vi "Out_On_N4_201.vi"(4 "Driver Name":T8, 6 "Error Code":T9, 7 "ADJUST":T6, 8 "error in":T7, 11 "DriverConnect in":T1={"InterfaceType"=enum."VISA", "OpenedSession"="", "InterfaceSettings"={"Interface"=enum."RS232", "EOS 4 read"=enum."LF (\\n)", "EOS 4 write"=enum."LF (\\n)", "TMO, ms"=10000, "Sett"=variant(cluster{"Baud Rate":u32, "Data Bits":u16, "Parity":u16, "Stop Bits":u16, "Flow Control":u16, "Eho":bool} {"Baud Rate"=75, "Data Bits"=0, "Parity"=0, "Stop Bits"=0, "Flow Control"=0, "Eho"=FALSE})}}) -> (0 "error out":T7, 3 "DriverConnect out":T1={"InterfaceType"=enum."VISA", "OpenedSession"="", "InterfaceSettings"={"Interface"=enum."RS232", "EOS 4 read"=enum."LF (\\n)", "EOS 4 write"=enum."LF (\\n)", "TMO, ms"=10000, "Sett"=variant(cluster{"Baud Rate":u32, "Data Bits":u16, "Parity":u16, "Stop Bits":u16, "Flow Control":u16, "Eho":bool} {"Baud Rate"=75, "Data Bits"=0, "Parity"=0, "Stop Bits"=0, "Flow Control"=0, "Eho"=FALSE})}})   [LabVIEW 2018]
uses:
  MOKO_LabViewLibrary/MokoLowLevel/MokoLowLovelControl/MLLC_ErrorCode.ctl
  MOKO_LabViewLibrary/MokoLowLevel/MokoLowLovelControl/MLLC_DriverName.ctl
  MOKO_LabViewLibrary/MokoLowLevel/MokoLowLovelControl/MLLC_Error.ctl
  MOKO_LabViewLibrary/MokoLowLevel/MokoLowLovelControl/MLLC_Delay.ctl
  MOKO_LabViewLibrary/MokoLowLevel/MokoLowLovelControl/MLLC_ConnectCluster.ctl
  MOKO_LabViewLibrary/MokoLowLevel/MokoLowLovelControl/MLLC_InterfaceType.ctl
  MOKO_LabViewLibrary/MokoLowLevel/MokoLowLovelControl/MLLC_OpenedSession.ctl
  MOKO_LabViewLibrary/MokoLowLevel/MokoLowLovelControl/MLLC_InterfaceSettings.ctl
  MOKO_LabViewLibrary/MokoLowLevel/MokoLowLovelControl/MLLC_InterfaceKind.ctl
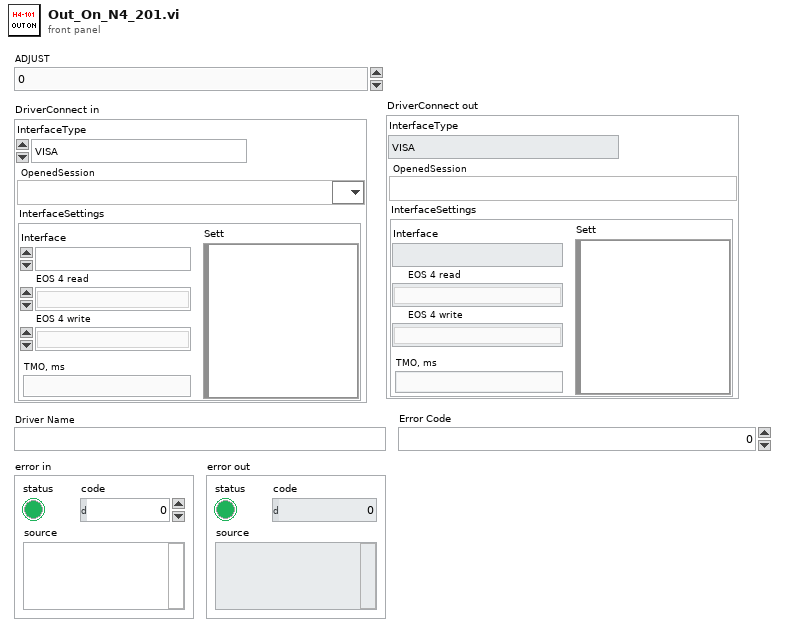
[diagram p1: front panel]
types:
  T1 = typedef "MLLC_ConnectCluster.ctl" = cluster{"InterfaceType":T2, "OpenedSession":T3, "InterfaceSettings":T4}
  T2 = typedef "MLLC_InterfaceType.ctl" = enum16{"VISA", "Prologix USB-GPIB"}
  T3 = typedef "MLLC_OpenedSession.ctl" = refnum<visa-resource-name>
  T4 = typedef "MLLC_InterfaceSettings.ctl" = cluster{"Interface":T5, "EOS 4 read":enum16{"Default (=EOS 4 write)", "CR (\\r)", "LF (\\n)", "None"}, "EOS 4 write":enum16{"CR+LF (\\r\\n)", "CR (\\r)", "LF (\\n)", "None"}, "TMO, ms":i32, "Sett":variant}
  T5 = typedef "MLLC_InterfaceKind.ctl" = enum16{"RS232", "GPIB", "USB", "Ethernet", "another"}
  T6 = typedef "MLLC_Delay.ctl" = dbl
  T7 = typedef "MLLC_Error.ctl" = errorcluster
  T8 = typedef "MLLC_DriverName.ctl" = string
  T9 = typedef "MLLC_ErrorCode.ctl" = u32
  T10 = enum16{"Нет симуляции", "В ручную", "Игнорировать"}
  T11 = typedef "MLLC_Response.ctl" = string
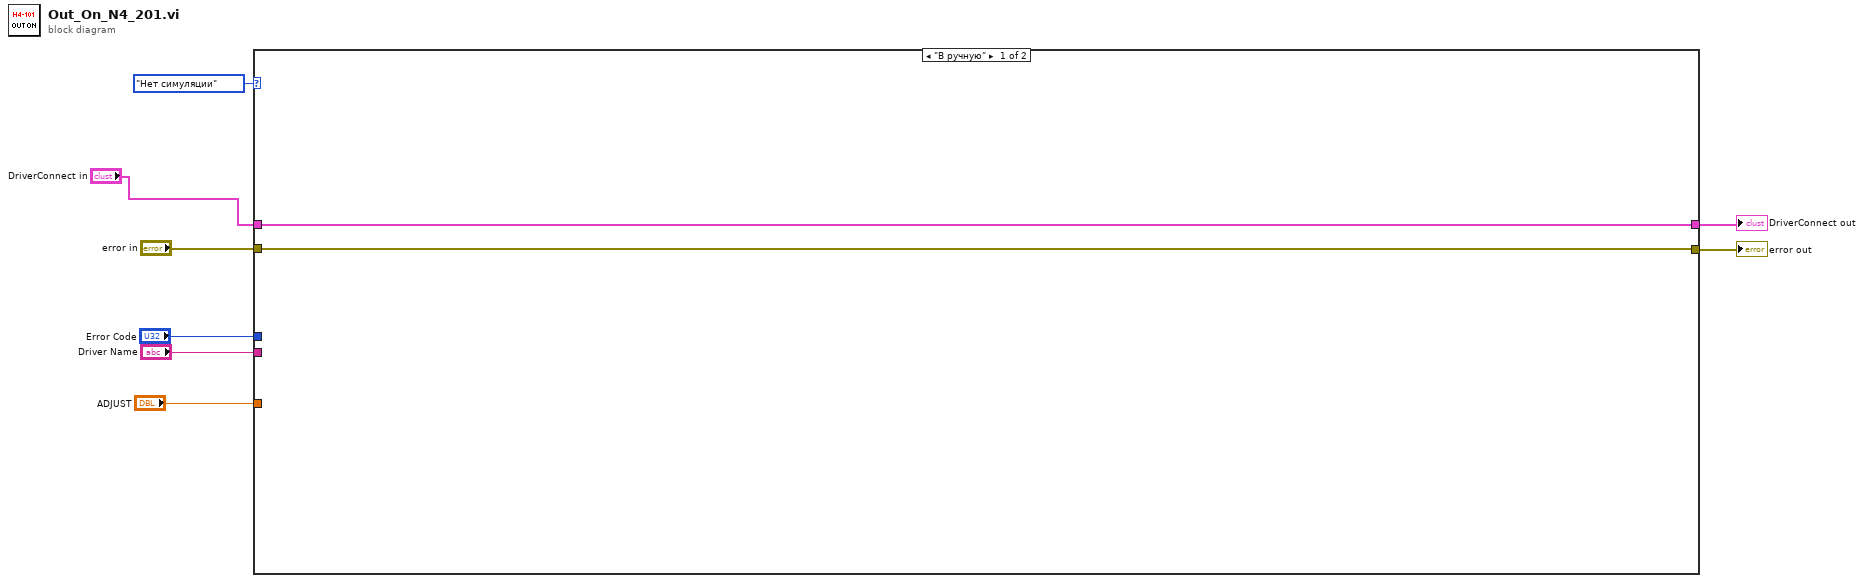
[diagram p0: block diagram]
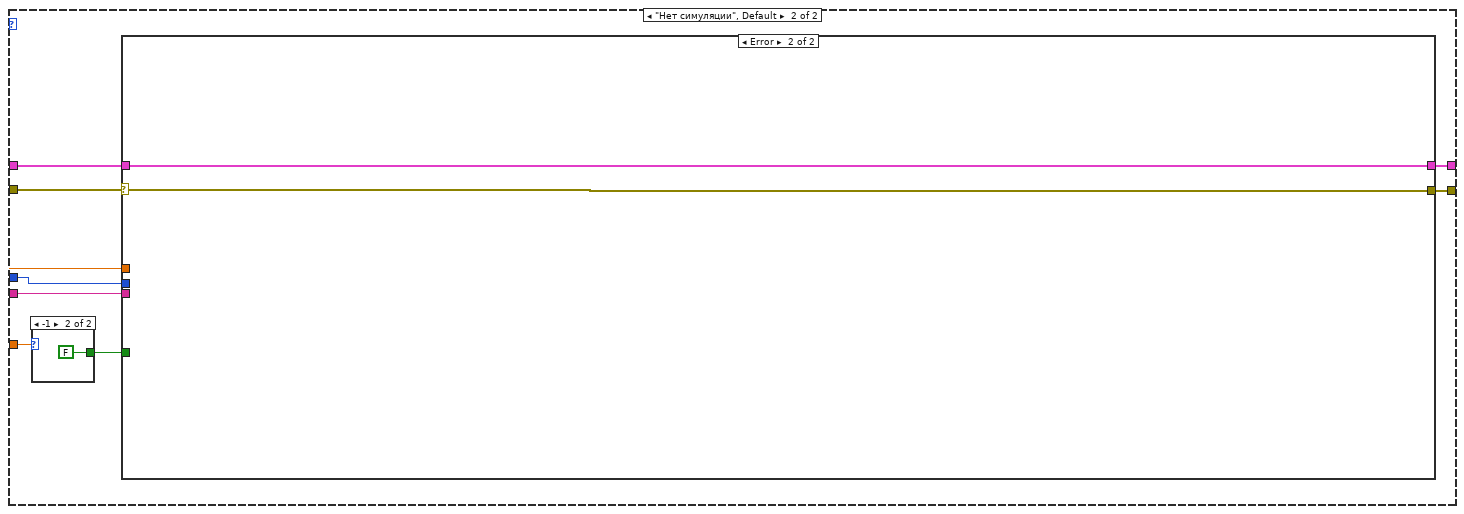
[diagram p2: hidden frame]
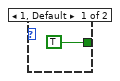
[diagram p3: hidden frame]
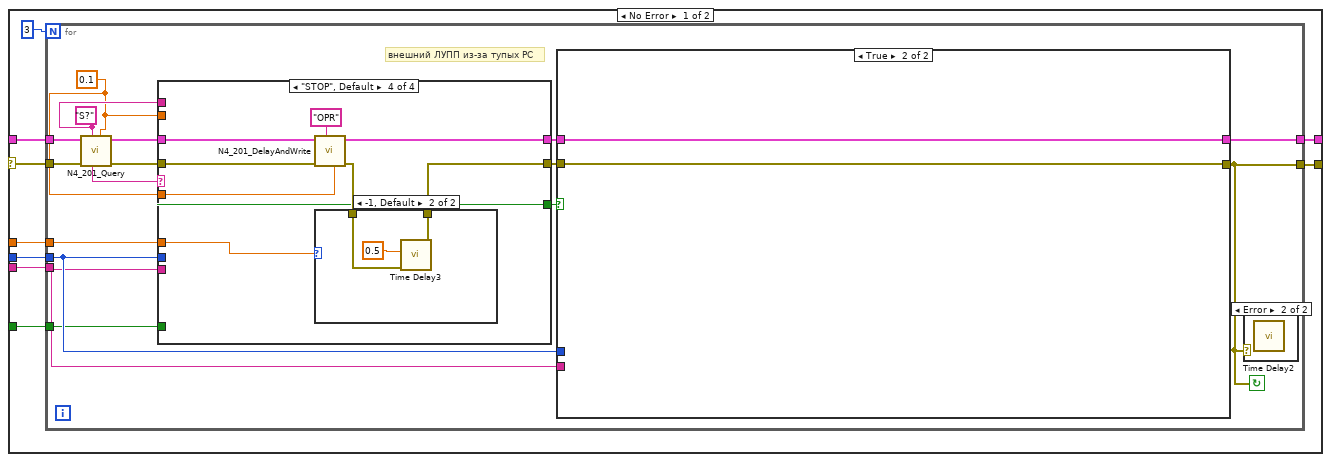
[diagram p4: hidden frame]
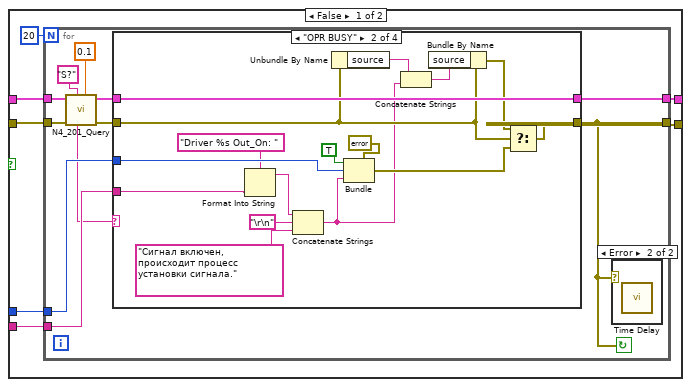
[diagram p6: hidden frame]
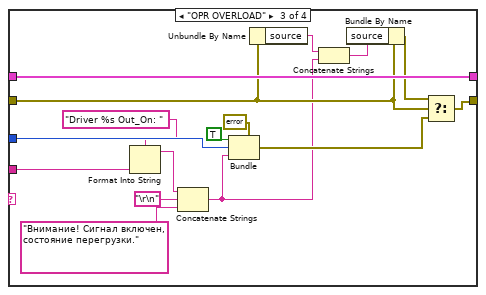
[diagram p8: hidden frame]
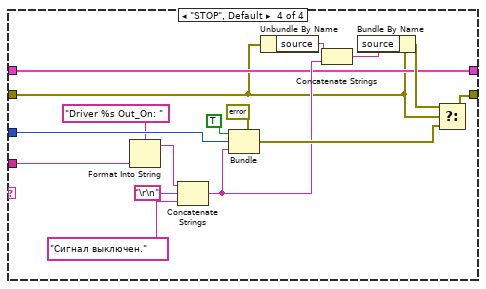
[diagram p9: hidden frame]
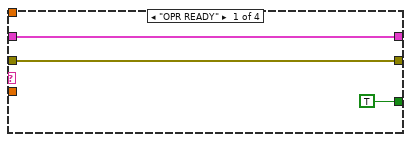
[diagram p11: hidden frame]
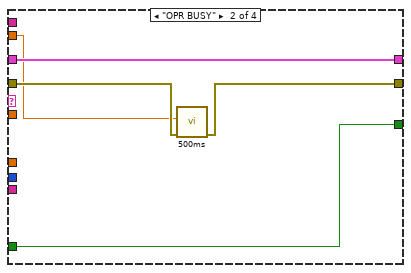
[diagram p12: hidden frame]
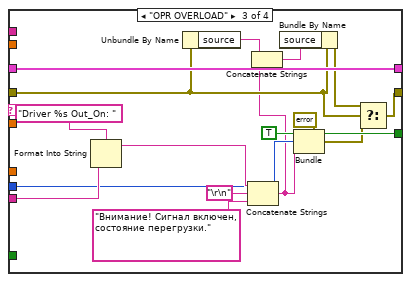
[diagram p13: hidden frame]
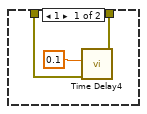
[diagram p14: hidden frame]
diagram:
  n1 = case shown="\"В ручную\"" T10."Нет симуляции" ("Simmulation") {
    tunnel: "DriverConnect in" -> [w10 w18]
    tunnel: "error in" -> [w9 w17]
    tunnel: "Error Code" -> [_ w16]
    tunnel: "Driver Name" -> [_ w15]
    tunnel: [w9 w14] -> w5
    tunnel: [w10 w13] -> w1
    tunnel: "ADJUST" -> [_ w11]
    frame "В ручную" {
    }
    frame "Нет симуляции", Default {
      n2 = case shown="-1" w11 {
        tunnel: [TRUE ("Status") FALSE ("Status")] -> w12
        frame 1, Default {
        }
        frame -1 {
        }
      }
      n3 = case shown="Error" w17 {
        selector: w17 -> [w22 w155]
        tunnel: w18 -> [w23 w156]
        tunnel: [w26 w156] -> w13
        tunnel: [w25 w155] -> w14
        tunnel: w15 -> [w28 _]
        tunnel: w16 -> [w29 _]
        tunnel: w12 -> [w27 _]
        tunnel: w11 -> [w21 _]
        frame No Error {
          n4 = for {
            N: 3 -> [_]
            tunnel: w29 -> [w39]
            tunnel: w28 -> [w38]
            tunnel: w27 -> [w37]
            tunnel: [w36] -> w26
            tunnel: [w33] -> w25
            tunnel: w23 -> [w35]
            tunnel: w22 -> [w34]
            tunnel: w21 -> [w30]
            stop <- w33 continue-if-true
            w31 = 0.1 ("Delay Time (s)")
            w32 = "S?" ("Error Query")
            # "внешний ЛУПП из-за тупых РС"
            n5 = call "N4_201_Query.vi"("Delay Befor (s)"=w31, "Command"=w32, "error in"=w34, "DriverConnect in"=w35) -> ("error out"=w43:T7, "DriverConnect out"=w44:T1, "Response"=w45:T11)  [unwired: 5 in]
            n6 = case shown="\"STOP\", Default" w45 {
              tunnel: w44 -> [w118 w122 w133 w147]
              tunnel: w43 -> [w117 w120 w127 w146]
              tunnel: [w118 w122 w133 w142] -> w42
              tunnel: [w117 w121 w125 w143] -> w40
              tunnel: w38 -> [_ _ w136 _]
              tunnel: w39 -> [_ _ w135 _]
              tunnel: w31 -> [_ _ _ w145]
              tunnel: [TRUE w123 w132 w141] -> w41
              tunnel: w37 -> [_ w123 _ w141]
              tunnel: w32 -> [_ _ _ _]
              tunnel: w31 -> [_ w119 _ _]
              tunnel: w30 -> [_ _ _ w140]
              frame "OPR READY" {
              }
              frame "OPR BUSY" {
                n7 = call "500ms"("error in (no error)"=w120, "Delay Time (s)"=w119) -> ("error out"=w121:errorcluster)  [unwired: 9 in]
              }
              frame "OPR OVERLOAD" {
                w132 = TRUE ("Status")
                n8 = Format Into String(format string="Driver %s Out_On: ", w136) -> (resulting string=w137:string)  [unwired: 2 in, 1 out]
                n9 = Unbundle By Name(w127) -> ("source"=w131:string)
                n10 = Concatenate Strings(w137, "\r\n", "Внимание! Сигнал включен, состояние перегрузки." ("string")) -> (w124:string)
                n11 = Concatenate Strings(w131, w124) -> (w130:string)
                n12 = Bundle By Name(cluster=w127, "source"=w130) -> (w126:T7)
                n13 = Bundle(cluster=errorcluster {"status"=FALSE, "code"=0, "source"=""} ("error out"), "status"=w132, "code"=w135, "source"=w124) -> (w128:errorcluster)
                n14 = Select(t=w126, s=w127, f=w128) -> (s? t:f=w125:T7)
              }
              frame "STOP", Default {
                n15 = call "N4_201_DelayAndWrite.vi"("Delay Befor (s)"=w145, "Command"="OPR" ("String"), "error in"=w146, "DriverConnect in"=w147) -> ("error out"=w144:T7, "DriverConnect out"=w142:T1)  [unwired: 6 in]
                n16 = case shown="-1, Default" w140 {
                  tunnel: w144 -> [w150 w154]
                  tunnel: [w149 w153] -> w143
                  frame 1 {
                    n17 = call "Time Delay4"("error in (no error)"=w150, "Delay Time (s)"=0.1) -> ("error out"=w149:errorcluster)  [unwired: 9 in]
                  }
                  frame -1, Default {
                    n18 = call "Time Delay3"("error in (no error)"=w154, "Delay Time (s)"=0.5) -> ("error out"=w153:errorcluster)  [unwired: 9 in]
                  }
                }
              }
            }
            n19 = case shown="True" w41 {
              tunnel: w42 -> [w52 w115]
              tunnel: [w49 w115] -> w36
              tunnel: [w48 w114] -> w33
              tunnel: w40 -> [w51 w114]
              tunnel: w39 -> [w47 _]
              tunnel: w38 -> [w46 _]
              frame False {
                n20 = for {
                  N: 20 -> [_]
                  tunnel: w52 -> [w61]
                  tunnel: w51 -> [w60]
                  tunnel: [w57] -> w49
                  tunnel: [w56] -> w48
                  tunnel: w47 -> [w55]
                  tunnel: w46 -> [w54]
                  stop <- w56 continue-if-true
                  n21 = call "N4_201_Query.vi"("Delay Befor (s)"=0.1 ("Delay Time (s)"), "Command"="S?" ("Error Query"), "error in"=w60, "DriverConnect in"=w61) -> ("error out"=w58:T7, "DriverConnect out"=w59:T1, "Response"=w53:T11)  [unwired: 5 in]
                  n22 = case shown="\"OPR BUSY\"" w53 {
                    tunnel: w59 -> [w65 w81 w90 w99]
                    tunnel: w58 -> [w64 w70 w83 w98]
                    tunnel: [w65 w81 w90 w99] -> w57
                    tunnel: [w64 w67 w86 w101] -> w56
                    tunnel: w54 -> [_ w75 w93 w109]
                    tunnel: w55 -> [_ w76 w92 w108]
                    frame "OPR READY" {
                    }
                    frame "OPR BUSY" {
                      n23 = Format Into String(format string="Driver %s Out_On: ", w75) -> (resulting string=w78:string)  [unwired: 2 in, 1 out]
                      n24 = Concatenate Strings(w78, "\r\n", "Сигнал включен, происходит процесс установки сигнала." ("string")) -> (w66:string)
                      n25 = Unbundle By Name(w70) -> ("source"=w73:string)
                      n26 = Bundle(cluster=errorcluster {"status"=FALSE, "code"=0, "source"=""} ("error out"), "status"=TRUE ("Status"), "code"=w76, "source"=w66) -> (w68:errorcluster)
                      n27 = Concatenate Strings(w73, w66) -> (w72:string)
                      n28 = Bundle By Name(cluster=w70, "source"=w72) -> (w71:T7)
                      n29 = Select(t=w71, s=w70, f=w68) -> (s? t:f=w67:T7)
                    }
                    frame "OPR OVERLOAD" {
                      n30 = Format Into String(format string="Driver %s Out_On: ", w93) -> (resulting string=w95:string)  [unwired: 2 in, 1 out]
                      n31 = Concatenate Strings(w95, "\r\n", "Внимание! Сигнал включен, состояние перегрузки." ("string")) -> (w82:string)
                      n32 = Bundle(cluster=errorcluster {"status"=FALSE, "code"=0, "source"=""} ("error out"), "status"=TRUE ("Status"), "code"=w92, "source"=w82) -> (w87:errorcluster)
                      n33 = Unbundle By Name(w83) -> ("source"=w84:string)
                      n34 = Concatenate Strings(w84, w82) -> (w89:string)
                      n35 = Bundle By Name(cluster=w83, "source"=w89) -> (w85:T7)
                      n36 = Select(t=w85, s=w83, f=w87) -> (s? t:f=w86:T7)
                    }
                    frame "STOP", Default {
                      n37 = Format Into String(format string="Driver %s Out_On: ", w109) -> (resulting string=w111:string)  [unwired: 2 in, 1 out]
                      n38 = Concatenate Strings(w111, "\r\n", "Сигнал выключен." ("string")) -> (w102:string)
                      n39 = Bundle(cluster=errorcluster {"status"=FALSE, "code"=0, "source"=""} ("error out"), "status"=TRUE ("Status"), "code"=w108, "source"=w102) -> (w103:errorcluster)
                      n40 = Unbundle By Name(w98) -> ("source"=w104:string)
                      n41 = Concatenate Strings(w104, w102) -> (w106:string)
                      n42 = Bundle By Name(cluster=w98, "source"=w106) -> (w105:T7)
                      n43 = Select(t=w105, s=w98, f=w103) -> (s? t:f=w101:T7)
                    }
                  }
                  n44 = case shown="Error" w56 {
                    frame No Error {
                    }
                    frame Error {
                      n45 = call "Time Delay"() -> ()  [unwired: 11 in, 1 out]
                    }
                  }
                }
              }
              frame True {
              }
            }
            n46 = case shown="Error" w33 {
              frame No Error {
              }
              frame Error {
                n47 = call "Time Delay2"() -> ()  [unwired: 11 in, 1 out]
              }
            }
          }
        }
        frame Error {
        }
      }
    }
  }
  "error out" <- w5
  "DriverConnect out" <- w1
